vi "Create.vi"(6 "Autostart (F)":bool, 7 "Param Type (Variant)":refnum<class>, 8 "error in (no error)":errorcluster, 10 "Result Type (Variant)":refnum<class>) -> (0 "error out":errorcluster, 3 "Promise":refnum<class "Promise.lvclass">)   [LabVIEW 2023, in "Promises.lvlib" / "Promise.lvclass"]
doc: "Creates a Promise that can be used in asynchronous code to return a result. Code that needs the result should first retrieve the Future with <b>Future.vi</b> and then use the <b>Wait.vi</b> of the Future to retrieve the result. Before calling <b>Wait.vi</b>, <b>Then.vi</b> can be called to chain Promises and perform many tasks in sequence once the previous tasks resolve.\n\nThe Promise can be immediately started and not wait for the input parameter by setting <b>Autostart</b> to true. When <b>Autostart</b> is true, the value passed in as the <b>Param Type</b> will be immediately send in as the Promise parameter."
uses:
  Promise.lvclass
  Result.ctl
  Result State.ctl
  Parameter Data.ctl
  Promise.lvclass/Promise.ctl
  Variant/Variant.lvclass
  Promises.lvlib
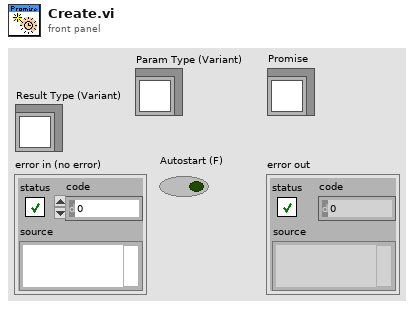
[diagram p1: front panel]
types:
  T1 = typedef "Promises.lvlib/Parameter Data.ctl" = cluster{"Parameter":refnum<class>}
  T2 = typedef "Promises.lvlib/Result.ctl" = cluster{"State":T3, "Value":refnum<class>}
  T3 = typedef "Promises.lvlib/Result State.ctl" = enum16{"Unset", "Error", "Success"}
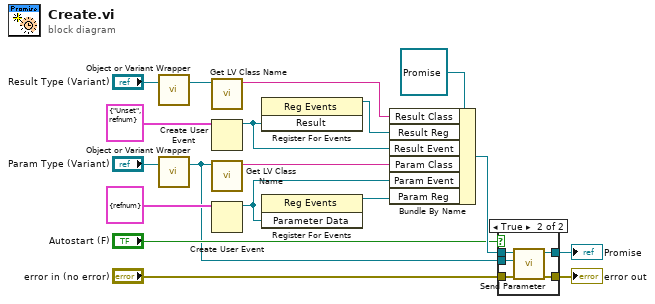
[diagram p0: block diagram]
diagram:
  n1 = call "Object or Variant Wrapper.vi"("LabVIEW Object"="Result Type (Variant)") -> ("Object or Variant Wrapper"=w2:refnum<class>)  [unwired: 6 in]
  n2 = call "Object or Variant Wrapper.vi"("LabVIEW Object"="Param Type (Variant)") -> ("Object or Variant Wrapper"=w1:refnum<class>)  [unwired: 6 in]
  n3 = call <vilib>:"Get LV Class Name.vi"("object"=w2) -> ("class name"=w6:string)  [unwired: 9 in, 1 out]
  n4 = Create User Event(user event datatype=T2 {"State"=enum."Unset", "Value"=refnum} ("Result")) -> (user event=w11:refnum<user-event>)  [unwired: 1 in, 1 out]
  n5 = call <vilib>:"Get LV Class Name.vi"("object"=w1) -> ("class name"=w18:string)  [unwired: 9 in, 1 out]
  n6 = Create User Event(user event datatype=T1 {"Parameter"=refnum} ("Parameter Data")) -> (user event=w9:refnum<user-event>)  [unwired: 1 in, 1 out]
  n7 = register-events(w11) -> (reference out=w7:refnum<event-registration>)  [unwired: 2 in, 1 out]
  n8 = register-events(w9) -> (reference out=w8:refnum<event-registration>)  [unwired: 2 in, 1 out]
  n9 = Bundle By Name(cluster=refnum<class "Promise.lvclass"> refnum ("Promise Type"), "Result Class"=w6, "Result Reg"=w7, "Result Event"=w11, "Param Class"=w18, "Param Event"=w9, "Param Reg"=w8) -> (w13:refnum<class "Promise.lvclass">)
  n10 = case shown="True" "Autostart (F)" {
    tunnel: w13 -> [w20 w25]
    tunnel: [w20 w24] -> w17
    tunnel: [w19 w23] -> w15
    tunnel: "error in (no error)" -> [w19 w22]
    tunnel: w1 -> [_ w21]
    frame False {
    }
    frame True {
      n11 = call "Send Parameter.vi"("error in (no error)"=w22, "Parameter"=w21, "Promise in"=w25) -> ("error out"=w23:errorcluster, "Promise out"=w24:refnum<class "Promise.lvclass">)  [unwired: 7 in]
    }
  }
  "error out" <- w15
  "Promise" <- w17
